vi "Tag Names.vi"(11 "State in":T1={"State"=enum."Idle", "Start Time"=timestamp(0 s since 1904-01-01), "Configuration"={"Cycle Period"=0.0, "PID 2 Parameters"={"Input Device"=enum."4-20mA", "Output Device"=enum."Default", "Setpoint"=0.0, "PID gains"={"proportional gain (Kc)"=0.0, "integral time (Ti, min)"=0.0, "derivative time (Td, min)"=100.0}, "output range"={"output low"=0.0, "output high"=1.0}}, "Manual Entry"=0.0, "Auto?"=TRUE, "4-20mA Input Settings"={"Input Channel "=0}, "4-20mA Out Settings"={"Output DAQ Task"=""}, "Input Channel Tag Name "=""}, "Current Time"=timestamp(0 s since 1904-01-01), "PID 1 Parameters"={"Setpoint"=0.0, "PID gains"={"proportional gain (Kc)"=1.0, "integral time (Ti, min)"=0.01, "derivative time (Td, min)"=0.0}}, "First Iteration"=FALSE, "Data"={"4-20mA Input"=0.0, "PID 2 Process Variable"=0.0, "PID 2 Output"=0.0, "4-20mA Output"=0.0}, "Process Name"="", "Pump On?"=enum."Off", "Input Error"=FALSE, "Output Error"=FALSE, "Log Started"=FALSE} {"Configuration"."PID 2 Parameters"."output range"."output low" format="%.2f"; "Configuration"."PID 2 Parameters"."output range"."output high" min=0.0 max=100.0 format="%.2f"; "Configuration"."PID 2 Parameters"."PID gains"."derivative time (Td, min)" format="%.3f"; "Configuration"."PID 2 Parameters"."PID gains"."integral time (Ti, min)" format="%.3f"; "Configuration"."PID 2 Parameters"."PID gains"."proportional gain (Kc)" format="%.3f"; "PID 1 Parameters"."PID gains"."derivative time (Td, min)" format="%.3f"; "PID 1 Parameters"."PID gains"."integral time (Ti, min)" format="%.3f"; "PID 1 Parameters"."PID gains"."proportional gain (Kc)" format="%.3f"}) -> (3 "4-20mA Module Tag Names":T6, 4 "All Boolean Tags":string[](array[string]), 5 "All  Numeric Tags":string[](array[string]))   [LabVIEW 2018, in "4-20mA Module.lvlib" / "4-20mA Module Engine.lvlib"]
uses:
  4-20mA Module Engine.lvlib
  Pressure Regulator/Controls/4-20mA Module Tag Names Cluster.ctl
  State Cluster.ctl
  State Enum.ctl
  Pressure Transmitter/Pressure Transmitter Device Settings.ctl
  Pressure Reg Module/Pressure Regulator Device Settings.ctl
  Measure Instrument/PID 1 Parameters Cluster.ctl
  Pressure Regulator/4-20mA Module.lvlib
  Pressure Transmitter/Pressure Transmitter Library.lvlib
  Pressure Reg Module/Pressure Regulator Library.lvlib
panel:
  out "PID 2 Out Tag":string
  # "Instrument Settings"
  # "Instrument Settings"
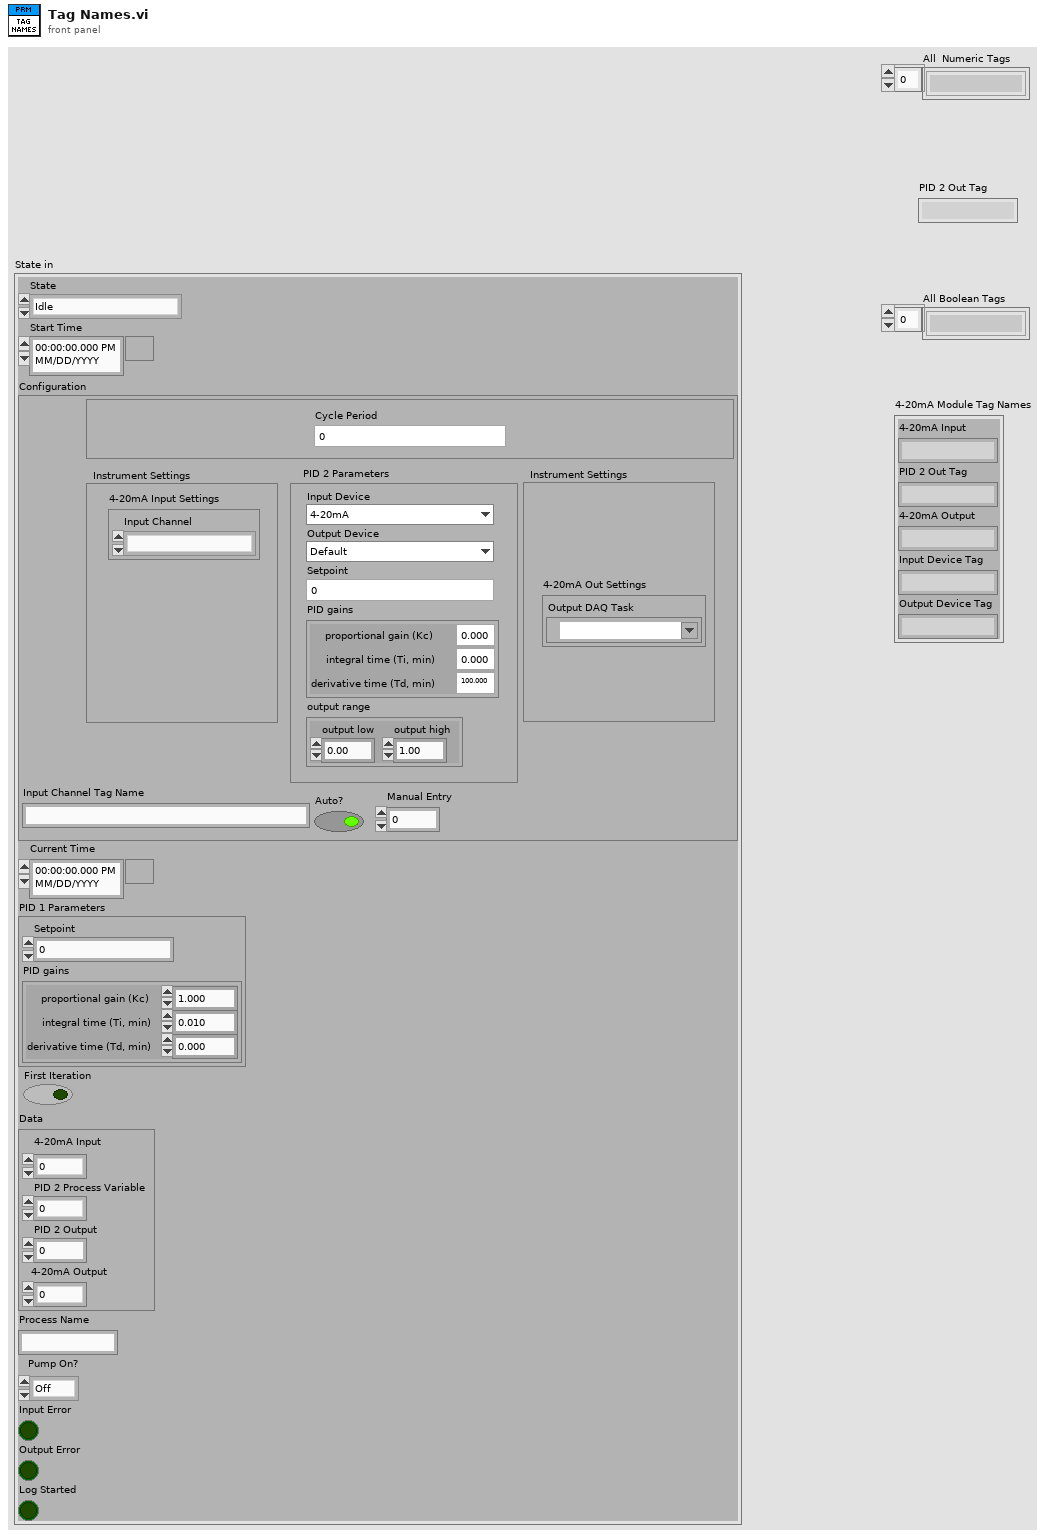
[diagram p1: front panel]
types:
  T1 = typedef "4-20mA Module.lvlib/4-20mA Module Engine.lvlib/State Cluster.ctl" = cluster{"State":T2, "Start Time":timestamp, "Configuration":cluster{"Cycle Period":dbl, "PID 2 Parameters":cluster{"Input Device":enum16{"Default", "4-20mA"}, "Output Device":enum16{"Default", "4-20mA"}, "Setpoint":dbl, "PID gains":cluster{"proportional gain (Kc)":dbl, "integral time (Ti, min)":dbl, "derivative time (Td, min)":dbl}, "output range":cluster{"output low":dbl, "output high":dbl}}, "Manual Entry":dbl, "Auto?":bool, "4-20mA Input Settings":T3, "4-20mA Out Settings":T4, "Input Channel Tag Name ":string}, "Current Time":timestamp, "PID 1 Parameters":T5, "First Iteration":bool, "Data":cluster{"4-20mA Input":dbl, "PID 2 Process Variable":dbl, "PID 2 Output":dbl, "4-20mA Output":dbl}, "Process Name":string, "Pump On?":enum16{"Off", "On", "Not Initialized"}, "Input Error":bool, "Output Error":bool, "Log Started":bool}
  T2 = typedef "4-20mA Module.lvlib/4-20mA Module Engine.lvlib/State Enum.ctl" = enum16{"Measuring", "Idle", "Paused"}
  T3 = typedef "Pressure Transmitter Library.lvlib/Pressure Transmitter Device Settings.ctl" = cluster{"Input Channel ":u16}
  T4 = typedef "Pressure Regulator Library.lvlib/Pressure Regulator Device Settings.ctl" = cluster{"Output DAQ Task":refnum<k21>}
  T5 = typedef "PID 1 Parameters Cluster.ctl" = cluster{"Setpoint":dbl, "PID gains":cluster{"proportional gain (Kc)":dbl, "integral time (Ti, min)":dbl, "derivative time (Td, min)":dbl}}
  T6 = typedef "4-20mA Module.lvlib/4-20mA Module Tag Names Cluster.ctl" = cluster{"4-20mA Input":string, "PID 2 Out Tag":string, "4-20mA Output":string, "Input Device Tag":string, "Output Device Tag":string}
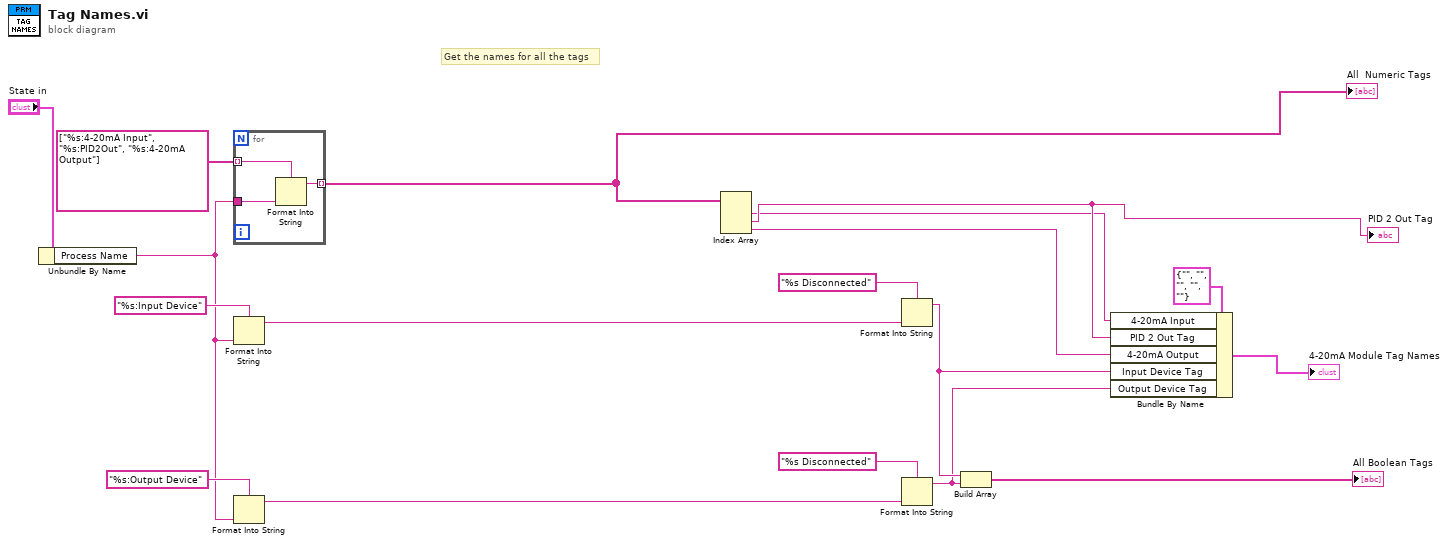
[diagram p0: block diagram]
diagram:
  # "Get the names for all the tags"
  n1 = Unbundle By Name("State in") -> ("Process Name"=w5:string)
  n2 = for {
    tunnel: string[] ["%s:4-20mA Input", "%s:PID2Out", "%s:4-20mA Output"] -> [w21] mode=indexing
    tunnel: w5 -> [w20]
    tunnel: [w19] -> w4 mode=indexing
    n3 = Format Into String(format string=w21, w20) -> (resulting string=w19:string)  [unwired: 2 in, 1 out]
  }
  "All  Numeric Tags" <- w4
  n4 = Format Into String(format string="%s:Input Device", w5) -> (resulting string=w15:string)  [unwired: 2 in, 1 out]
  n5 = Format Into String(format string="%s:Output Device", w5) -> (resulting string=w14:string)  [unwired: 2 in, 1 out]
  n6 = Index Array(array=w4) -> (element #1=w2:string, element #2=w3:string, element #3=w1:string)  [unwired: 3 in]
  "PID 2 Out Tag" <- w3
  n7 = Format Into String(format string="%s Disconnected", w15) -> (resulting string=w8:string)  [unwired: 2 in, 1 out]
  n8 = Format Into String(format string="%s Disconnected", w14) -> (resulting string=w7:string)  [unwired: 2 in, 1 out]
  n9 = Build Array(w8, w7) -> (→"All Boolean Tags":string[])
  n10 = Bundle By Name(cluster=T6 {"4-20mA Input"="", "PID 2 Out Tag"="", "4-20mA Output"="", "Input Device Tag"="", "Output Device Tag"=""} ("Feed Module Tag Names"), "4-20mA Input"=w2, "PID 2 Out Tag"=w3, "4-20mA Output"=w1, "Input Device Tag"=w8, "Output Device Tag"=w7) -> (→"4-20mA Module Tag Names":T6)
